vi "Proc Strain Channel.vi"(6 "channel name":string="p", 7 "offset duration":dbl=0.005 format="%#_6ps", 8 "error in (no error)":errorcluster, 9 "group name in":string="p", 10 "tdms file":refnum<k34>, 11 "Strain Logger in":refnum<class "Strain Logger.lvclass">) -> (0 "error out":errorcluster, 1 "Parameters":dbl[](array[numeric]), 2 "tdms file out":refnum<k34>, 3 "Strain Logger out":refnum<class "Strain Logger.lvclass">, 4 "Max time":dbl)   [LabVIEW 2024, in "Strain Logger.lvclass"]
uses:
  Strain Logger.lvclass
panel:
  out "Max value":dbl
  out "Waveform Graph":waveform(dbl)[](graph)
  # "Start\nEnd\nMax\nStreach\nTime"
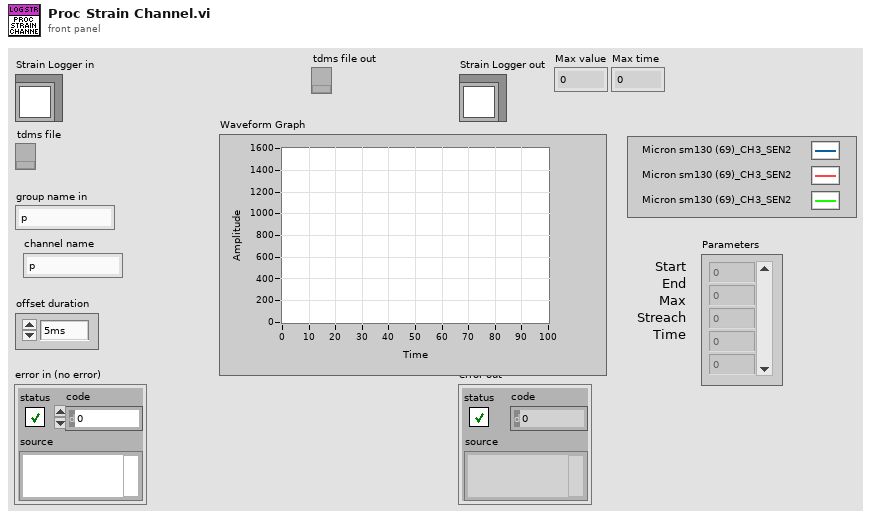
[diagram p1: front panel]
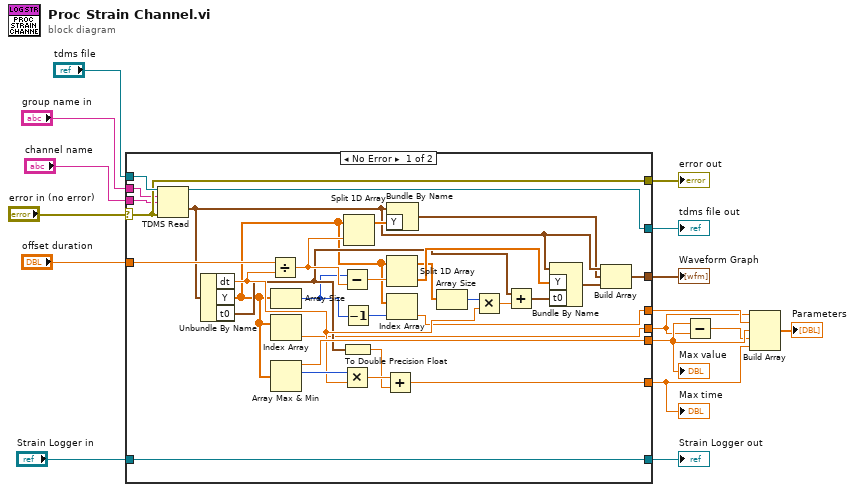
[diagram p0: block diagram]
diagram:
  n1 = case shown="No Error" "error in (no error)" {
    selector: "error in (no error)" -> [w44 w50]
    tunnel: [w44 w50] -> w15
    tunnel: [w47 w49] -> w13
    tunnel: "Strain Logger in" -> [w47 w49]
    tunnel: "tdms file" -> [w46 w48]
    tunnel: [w45 w48] -> w11
    tunnel: "channel name" -> [w42 _]
    tunnel: "group name in" -> [w43 _]
    tunnel: "offset duration" -> [w41 _]
    tunnel: [w29 _] -> w7
    tunnel: [w28 _] -> w3
    tunnel: [w22 _] -> w4
    tunnel: [w19 _] -> w2
    tunnel: [w18 _] -> w6
    frame No Error {
      n2 = TDMS Read(0:w46, 5:w43, 7:w42, 11:w44) -> (4:w45:refnum<k34>, 10:w32:waveform(dbl))  [unwired: 4 in, 4 out]
      n3 = Unbundle By Name(w32) -> ("dt"=w26:dbl, "Y"=w17:dbl[], "t0"=w25:timestamp)
      n4 = Divide(x=w41, y=w26) -> (x/y=w40:dbl)
      n5 = Array Size(array=w17) -> (size(s)=w21:i32)
      n6 = Index Array(array=w17) -> (element=w19:dbl)  [unwired: 1 in]
      n7 = Array Max & Min(array=w17) -> (max value=w28:dbl, max index (indices)=w27:i32)  [unwired: 2 out]
      n8 = Subtract(x=w21, y=w40) -> (x-y=w39:dbl)
      n9 = Multiply(x=w27, y=w26) -> (x*y=w24:dbl)
      n10 = Decrement(x=w21) -> (x-1=w20:i32)
      n11 = To Double Precision Float(number=w25) -> (double precision float=w23:dbl)
      n12 = Split 1D Array(array=w17, index=w40) -> (first subarray=w38:dbl[])  [unwired: 1 out]
      n13 = Add(x=w24, y=w23) -> (x+y=w22:dbl)
      n14 = Bundle By Name(cluster=w32, "Y"=w38) -> (w31:waveform(dbl))
      n15 = Split 1D Array(array=w17, index=w39) -> (first subarray=w36:dbl[], second subarray=w37:dbl[])
      n16 = Index Array(array=w17, index=w20) -> (element=w18:dbl)
      n17 = Array Size(array=w36) -> (size(s)=w35:i32)
      n18 = Multiply(x=w35, y=w26) -> (x*y=w34:dbl)
      n19 = Add(x=w25, y=w34) -> (x+y=w33:timestamp)
      n20 = Bundle By Name(cluster=w32, "Y"=w37, "t0"=w33) -> (w30:waveform(dbl))
      n21 = Build Array(w32, w31, w30) -> (w29:waveform(dbl)[])
    }
    frame Error {
    }
  }
  "error out" <- w15
  "Strain Logger out" <- w13
  "tdms file out" <- w11
  "Waveform Graph" <- w7
  "Max value" <- w3
  "Max time" <- w4
  n22 = Subtract(x=w3, y=w2) -> (x-y=w1:dbl)
  n23 = Build Array(w2, w6, w3, w1, w4) -> (→"Parameters":dbl[])
